vi "create io files.vi"(11 "path":path) -> (0 "interrupts.c":string, 2 "void init_ios(void)":string, 3 "defines":string)   [LabVIEW 2010]
uses:
  read_excel_values.llb/GetXL_CellValues_2D_String.vi
panel:
  out "error out":errorcluster
  # "Type: U8, I8, U16, I16, U32, I32, U64, I64, FLOAT"
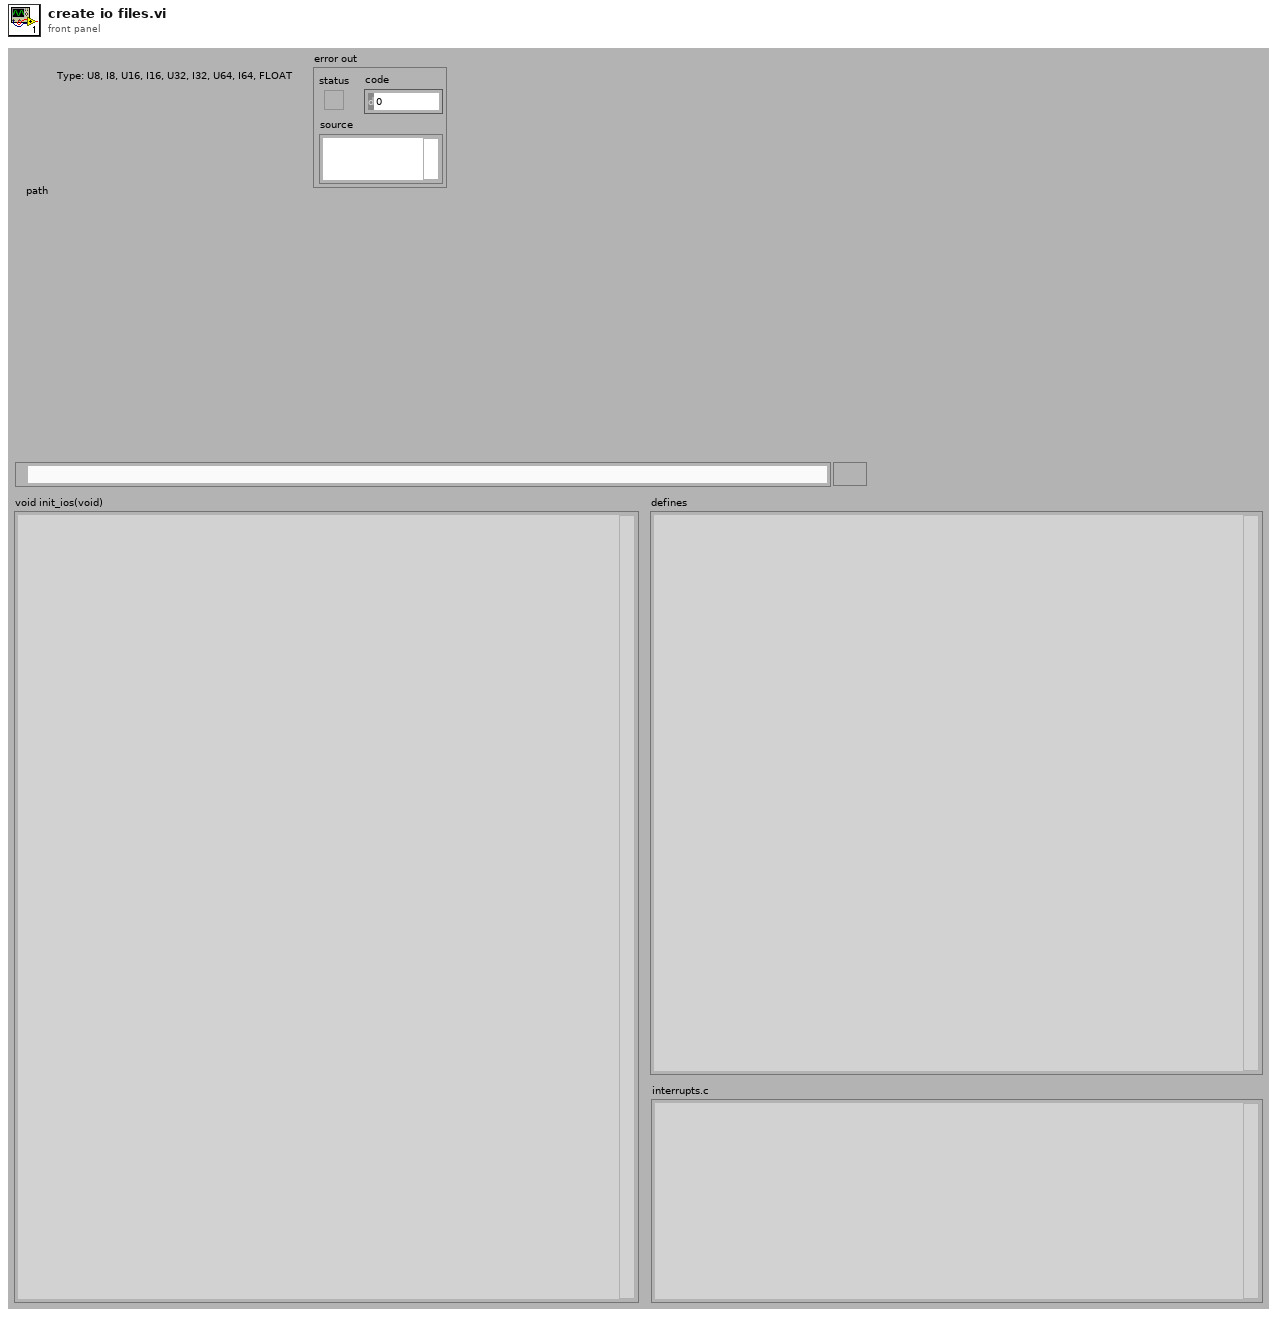
[diagram p1: front panel]
types:
  T1 = cluster{"Excel._Application":refnum<k7>, "Workbooks":refnum<k7>}
  T2 = cluster{"Excel._Application":refnum<k7>, "Workbooks":refnum<k7>, "Open":refnum<k7>}
  T3 = cluster{"Excel._Application":refnum<k7>, "Workbooks":refnum<k7>, "Open":refnum<k7>, "Worksheets":refnum<k7>, "Excel._Worksheet":refnum<k7>}
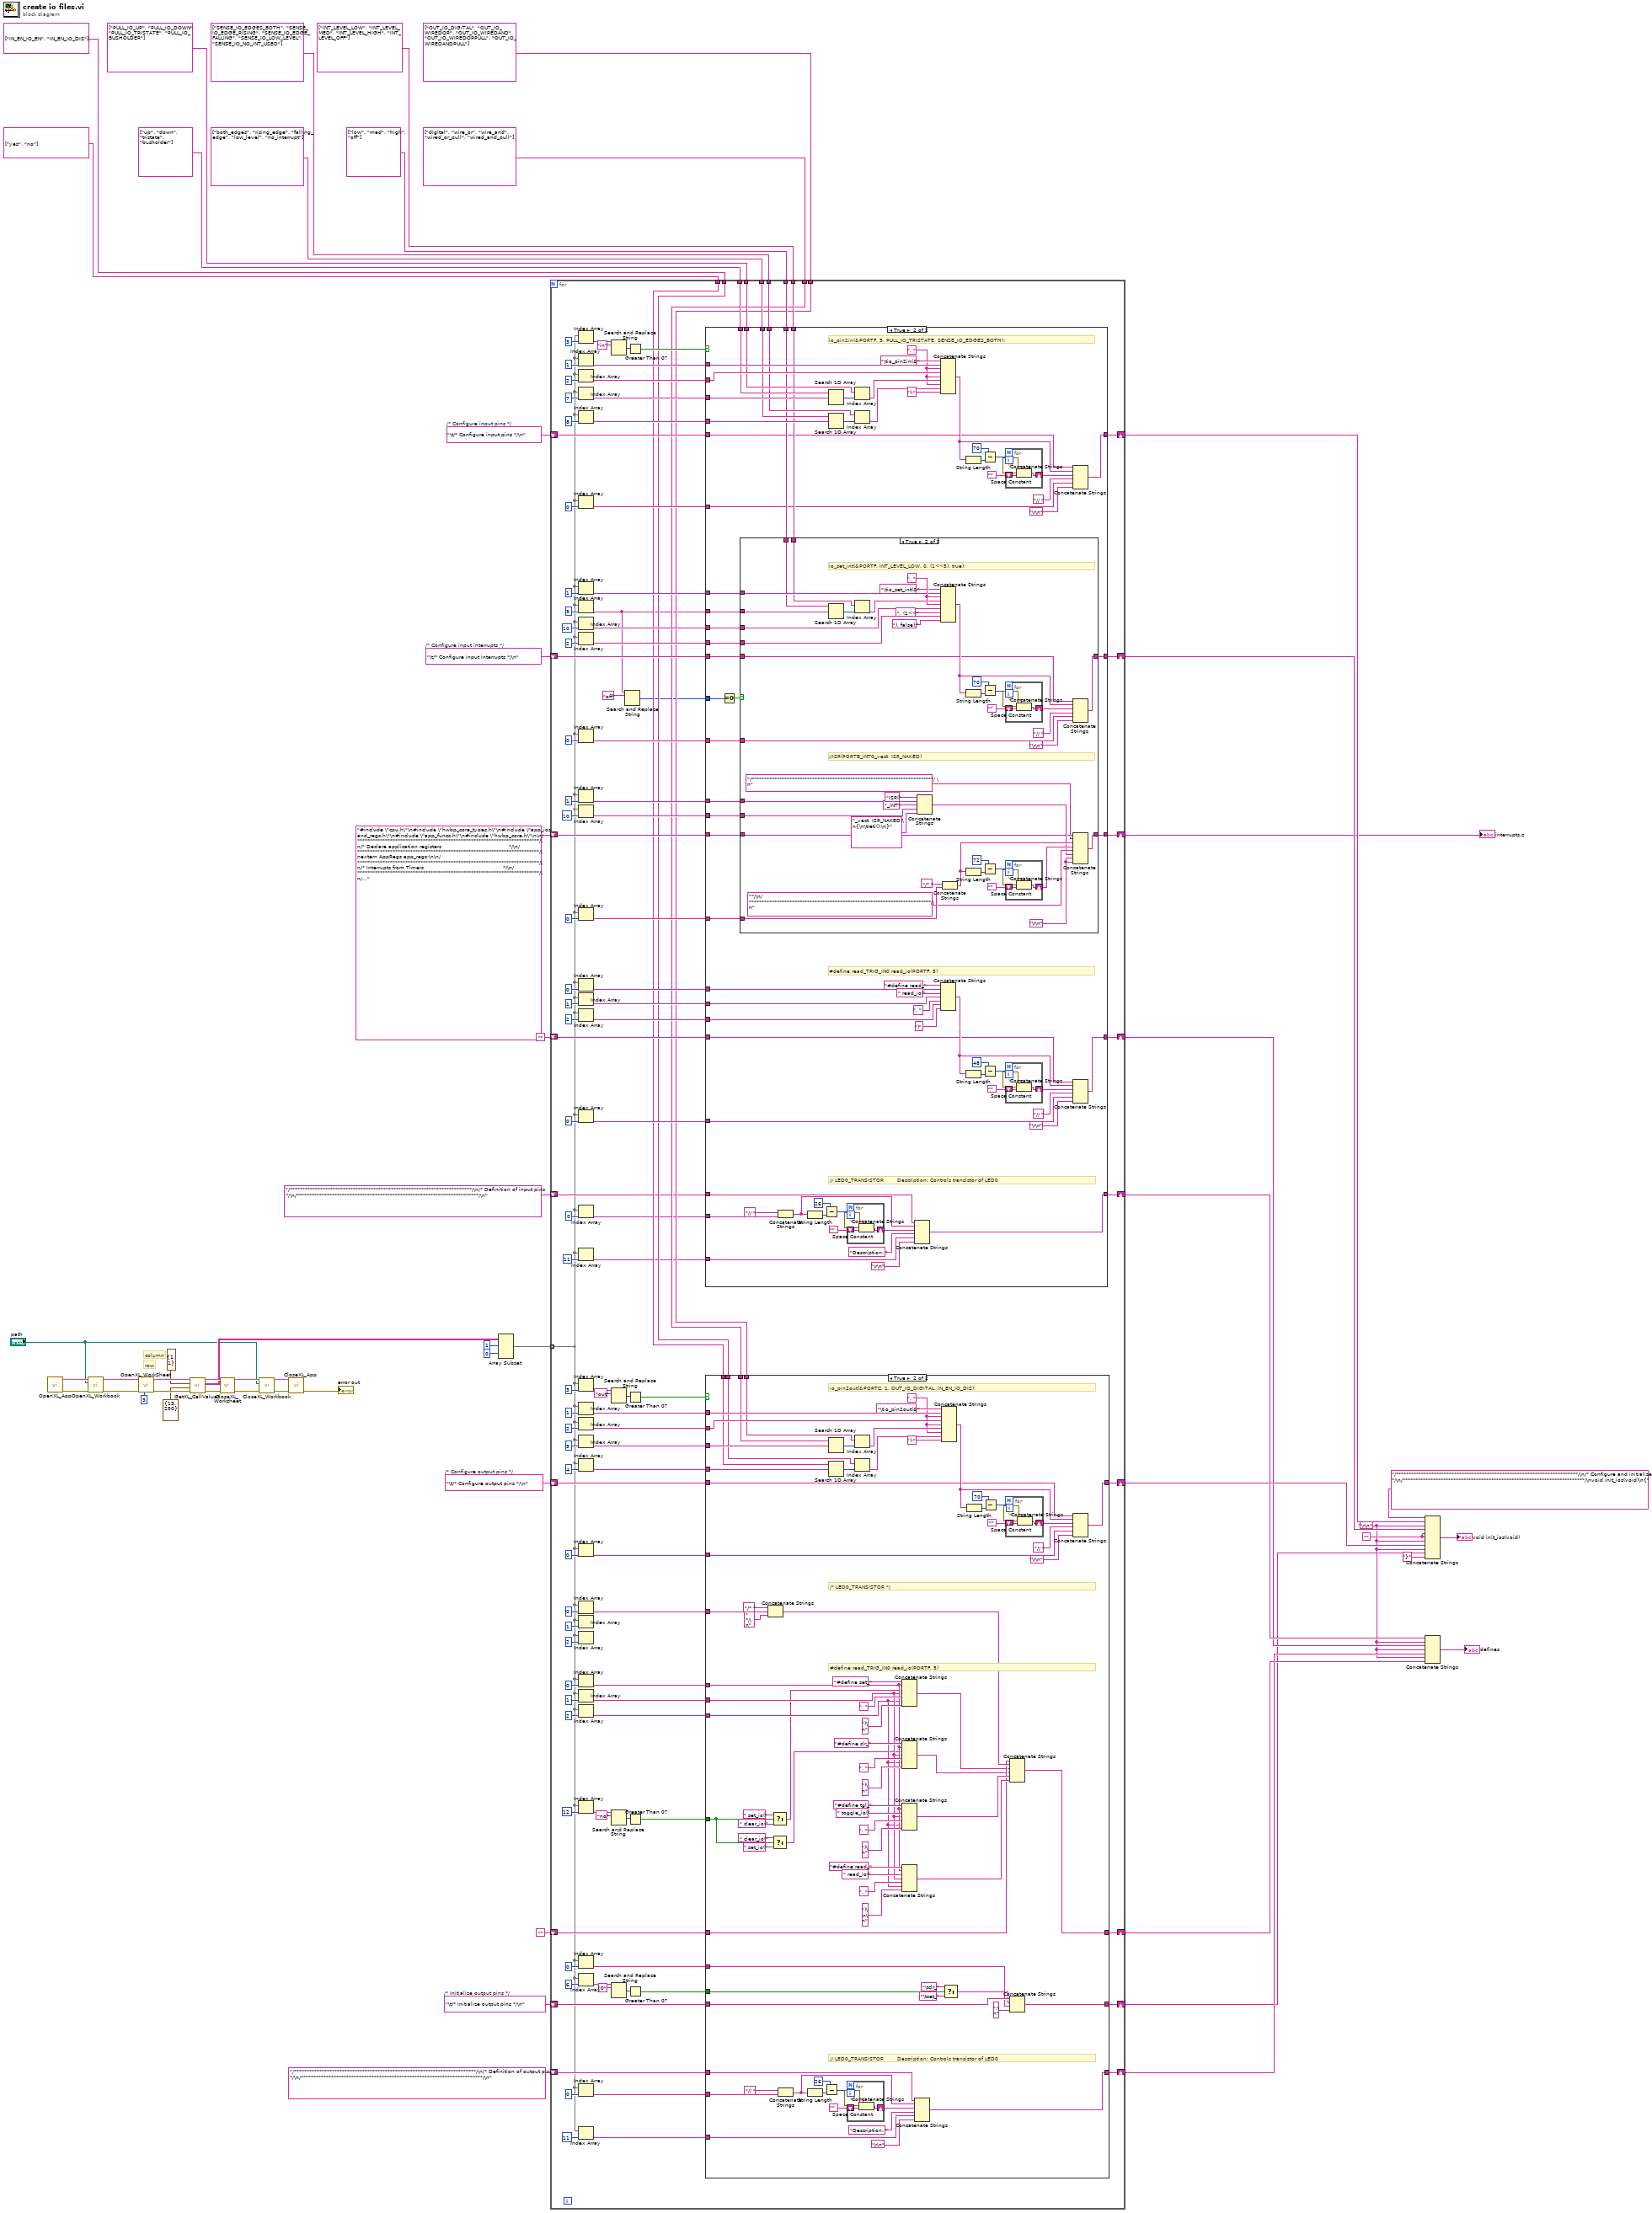
[diagram p0: block diagram]
diagram:
  w1 = ""
  w7 = "\t/* Configure input interrupts */\n"  # /* Configure input interrupts */
  w8 = "\t/* Configure output pins */\n"  # /* Configure output pins */
  w9 = "\t/* Configure input pins */\n"  # /* Configure input pins */
  w10 = "\t/* Initialize output pins */\n"  # /* Initialize output pins */
  w12 = "\r\n"
  # "row"
  # "column"
  n1 = call "OpenXL_App.vi"() -> ("error out"=w47:errorcluster, "Refnum Cluster"=w48:T1)  [unwired: 10 in]
  n2 = call "OpenXL_Workbook.vi"("error in"=w47, "path"="path", "Refnum Cluster In"=w48) -> ("error out"=w33:errorcluster, "Refnum Cluster Out"=w36:T2)  [unwired: 7 in]
  n3 = call "OpenXL_WorkSheet.vi"("Sheet"=3, "error in (no error)"=w33, "Refnum Cluster In"=w36) -> ("error out"=w54:errorcluster, "Refnum Cluster Out"=w55:T3)  [unwired: 7 in]
  n4 = call-poly "GetXL_CellValues.vi"("error in"=w54, "End"=cluster{"Column":i32, "Row":i32} {"Column"=13, "Row"=250}, "Start"=cluster{"Column":i32, "Row":i32} {"Column"=1, "Row"=1}, "Refnum Cluster In"=w55) -> ("error out"=w45:errorcluster, "data"=w40:string[][], "Refnum Cluster Out"=w46:T3)  [unwired: 5 in]
  n5 = call "CloseXL_Worksheet.vi"("error in (no error)"=w45, "Refnum Cluster In"=w46) -> ("error out"=w43:errorcluster, "Refnum Cluster Out"=w44:T2)  [unwired: 8 in]
  n6 = call "CloseXL_Workbook.vi"("error in (no error)"=w43, "path"="path", "Refnum Cluster In"=w44) -> ("error out"=w52:errorcluster, "Refnum Cluster Out"=w53:T1)  [unwired: 7 in]
  n7 = call "CloseXL_App.vi"("error in (no error)"=w52, "Refnum Cluster In"=w53) -> ("error out"=→"error out":errorcluster)  [unwired: 9 in]
  n8 = Array Subset(array=w40, index (row)=1 ("index"), index (col)=0 ("index")) -> (w37:string[][])  [unwired: 2 in]
  n9 = for {
    tunnel: w37 -> [w63] mode=indexing
    tunnel: string[] ["both_edges", "rising_edge", "falling_edge", "low_level", "no_interrupt"] -> [w155]
    tunnel: string[] ["up", "down", "tristate", "busholder"] -> [w159]
    shift-right: [w152] -> w23
    shift-left: w9 -> [w153]
    tunnel: string[] ["yes", "no"] -> [w95]
    tunnel: string[] ["IN_EN_IO_EN", "IN_EN_IO_DIS"] -> [w94]
    tunnel: string[] ["PULL_IO_UP", "PULL_IO_DOWN", "PULL_IO_TRISTATE", "PULL_IO_BUSHOLDER"] -> [w158]
    tunnel: string[] ["SENSE_IO_EDGES_BOTH", "SENSE_IO_EDGE_RISING", "SENSE_IO_EDGE_FALLING", "SENSE_IO_LOW_LEVEL", "SENSE_IO_NO_INT_USED"] -> [w154]
    tunnel: string[] ["low", "med", "high", "off"] -> [w142]
    tunnel: string[] ["INT_LEVEL_LOW", "INT_LEVEL_MED", "INT_LEVEL_HIGH", "INT_LEVEL_OFF"] -> [w141]
    tunnel: string[] ["digital", "wire_or", "wire_and", "wired_or_pull", "wired_and_pull"] -> [w92]
    tunnel: string[] ["OUT_IO_DIGITAL", "OUT_IO_WIREDOR", "OUT_IO_WIREDAND", "OUT_IO_WIREDORPULL", "OUT_IO_WIREDANDPULL"] -> [w93]
    shift-right: [w151] -> w24
    shift-left: w7 -> [w150]
    shift-right: [w129] -> w2
    shift-left: "#include \"cpu.h\"\n#include \"hwbp_core_types.h\"\n#include \"app_ios_and_regs.h\"\n#include \"app_funcs.h\"\n#include \"hwbp_core.h\"\n\n/************************************************************************/\n/* Declare application registers                                        */\n/************************************************************************/\nextern AppRegs app_regs;\n\n/************************************************************************/\n/* Interrupts from Timers                                               */\n/************************************************************************/\n// ISR(TCC0_OVF_vect, ISR_NAKED)\n// ISR(TCD0_OVF_vect, ISR_NAKED)\n// ISR(TCE0_OVF_vect, ISR_NAKED)\n// ISR(TCF0_OVF_vect, ISR_NAKED)\n// \n// ISR(TCC0_CCA_vect, ISR_NAKED)\n// ISR(TCD0_CCA_vect, ISR_NAKED)\n// ISR(TCE0_CCA_vect, ISR_NAKED)\n// ISR(TCF0_CCA_vect, ISR_NAKED)\n// \n// ISR(TCD1_OVF_vect, ISR_NAKED)\n// \n// ISR(TCD1_CCA_vect, ISR_NAKED)\n\n" -> [w130]
    shift-right: [w128] -> w14
    shift-left: "" -> [w127]
    shift-right: [w110] -> w19
    shift-left: w8 -> [w109]
    shift-right: [w89] -> w13
    shift-left: "/************************************************************************/\n/* Definition of output pins                                            */\n/************************************************************************/\n" -> [w88]
    shift-right: [w80] -> w11
    shift-left: "" -> [w87]
    shift-right: [w77] -> w15
    shift-left: "/************************************************************************/\n/* Definition of input pins                                             */\n/************************************************************************/\n" -> [w74]
    shift-right: [w72] -> w5
    shift-left: w10 -> [w71]
    n10 = Index Array(array=w63, index=3) -> (element=w168:string)
    n11 = Index Array(array=w63, index=1) -> (element=w164:string)
    n12 = Index Array(array=w63, index=2) -> (element=w162:string)
    n13 = Index Array(array=w63, index=7) -> (element=w160:string)
    n14 = Index Array(array=w63, index=8) -> (element=w156:string)
    n15 = Index Array(array=w63, index=0) -> (element=w135:string)
    n16 = Index Array(array=w63, index=1) -> (element=w144:string)
    n17 = Index Array(array=w63, index=9) -> (element=w58:string)
    n18 = Index Array(array=w63, index=10) -> (element=w149:string)
    n19 = Index Array(array=w63, index=2) -> (element=w146:string)
    n20 = Index Array(array=w63, index=0) -> (element=w134:string)
    n21 = Index Array(array=w63, index=1) -> (element=w139:string)
    n22 = Index Array(array=w63, index=10) -> (element=w137:string)
    n23 = Index Array(array=w63, index=0) -> (element=w131:string)
    n24 = Index Array(array=w63, index=0) -> (element=w122:string)
    n25 = Index Array(array=w63, index=1) -> (element=w124:string)
    n26 = Index Array(array=w63, index=2) -> (element=w119:string)
    n27 = Index Array(array=w63, index=0) -> (element=w126:string)
    n28 = Index Array(array=w63, index=3) -> (element=w98:string)
    n29 = Index Array(array=w63, index=1) -> (element=w102:string)
    n30 = Index Array(array=w63, index=2) -> (element=w104:string)
    n31 = Index Array(array=w63, index=5) -> (element=w106:string)
    n32 = Index Array(array=w63, index=4) -> (element=w108:string)
    n33 = Index Array(array=w63, index=0) -> (element=w112:string)
    n34 = Index Array(array=w63, index=0) -> (element=w116:string)
    n35 = Index Array(array=w63, index=1) -> ()  [unwired: 1 out]
    n36 = Index Array(array=w63, index=2) -> ()  [unwired: 1 out]
    n37 = Index Array(array=w63, index=0) -> (element=w84:string)
    n38 = Index Array(array=w63, index=1) -> (element=w86:string)
    n39 = Index Array(array=w63, index=2) -> (element=w81:string)
    n40 = Index Array(array=w63, index=12) -> (element=w60:string)
    n41 = Index Array(array=w63, index=0) -> (element=w65:string)
    n42 = Index Array(array=w63, index=6) -> (element=w68:string)
    n43 = Index Array(array=w63, index=0) -> (element=w90:string)
    n44 = Index Array(array=w63, index=11) -> (element=w113:string)
    n45 = Index Array(array=w63, index=0) -> (element=w76:string)
    n46 = Index Array(array=w63, index=11) -> (element=w75:string)
    n47 = Search and Replace String(input string=w168, search string="in") -> (number of replacements=w166:i32)  [unwired: 6 in, 3 out]
    n48 = Search and Replace String(input string=w98, search string="out") -> (number of replacements=w100:i32)  [unwired: 6 in, 3 out]
    n49 = Search and Replace String(input string=w60, search string="no") -> (number of replacements=w62:i32)  [unwired: 6 in, 3 out]
    n50 = Search and Replace String(input string=w68, search string="0") -> (number of replacements=w69:i32)  [unwired: 6 in, 3 out]
    n51 = Search and Replace String(input string=w58, search string="off") -> (number of replacements=w56:i32)  [unwired: 6 in, 3 out]
    n52 = Greater Than 0?(x=w166) -> (x > 0?=w165:bool)
    n53 = Greater Than 0?(x=w100) -> (x > 0?=w101:bool)
    n54 = Greater Than 0?(x=w62) -> (x > 0?=w59:bool)
    n55 = Greater Than 0?(x=w69) -> (x > 0?=w67:bool)
    n56 = case shown="True" w165 {
      tunnel: w164 -> [_ w338]
      tunnel: w162 -> [_ w337]
      tunnel: w160 -> [_ w335]
      tunnel: w159 -> [_ w334]
      tunnel: w158 -> [_ w333]
      tunnel: w156 -> [_ w329]
      tunnel: w155 -> [_ w328]
      tunnel: w154 -> [_ w327]
      tunnel: w153 -> [w266 w306]
      tunnel: [w266 w307] -> w152
      tunnel: w144 -> [_ w323]
      tunnel: w146 -> [_ w319]
      tunnel: w58 -> [_ w324]
      tunnel: w149 -> [_ w320]
      tunnel: w150 -> [w265 w303]
      tunnel: [w265 w304] -> w151
      tunnel: w142 -> [_ w322]
      tunnel: w141 -> [_ w321]
      tunnel: w139 -> [_ w318]
      tunnel: w137 -> [_ w317]
      tunnel: w135 -> [_ w309]
      tunnel: w134 -> [_ w305]
      tunnel: w130 -> [w264 w302]
      tunnel: [w264 w301] -> w129
      tunnel: w131 -> [_ w300]
      tunnel: w122 -> [_ w287]
      tunnel: w124 -> [_ w288]
      tunnel: w127 -> [w263 w289]
      tunnel: [w263 w290] -> w128
      tunnel: w126 -> [_ w297]
      tunnel: w119 -> [_ w284]
      tunnel: [w262 w272] -> w77
      tunnel: w76 -> [_ w271]
      tunnel: w75 -> [_ w270]
      tunnel: w74 -> [w262 w269]
      tunnel: w56 -> [_ w267]
      frame False {
      }
      frame True {
        w331 = ", " ("string")
        # "// LED0_TRANSISTOR        Description: Controls transistor of LED0"
        # "#define read_TRIG_IN0 read_io(PORTF, 5)"
        # "io_pin2in(&PORTF, 5, PULL_IO_TRISTATE, SENSE_IO_EDGES_BOTH);"
        n57 = Equal To 0?(x=w267) -> (x = 0?=w268:bool)
        n58 = case shown="True" w268 {
          tunnel: w324 -> [_ w382]
          tunnel: w323 -> [_ w380]
          tunnel: w322 -> [_ w378]
          tunnel: w321 -> [_ w377]
          tunnel: w320 -> [_ w375]
          tunnel: w319 -> [_ w373]
          tunnel: w318 -> [_ w368]
          tunnel: w317 -> [_ w367]
          tunnel: w305 -> [_ w365]
          tunnel: [w341 w357] -> w304
          tunnel: w303 -> [w341 w356]
          tunnel: w302 -> [w340 w343]
          tunnel: [w340 w355] -> w301
          tunnel: w300 -> [_ w348]
          frame False {
          }
          frame True {
            w344 = "\r\n"
            w383 = ", " ("string")
            # "//ISR(PORTB_INT0_vect, ISR_NAKED)"
            # "io_set_int(&PORTF, INT_LEVEL_LOW, 0, (1<<5), true);"
            n59 = Search 1D Array(1D array=w378, element=w382) -> (index of element=w381:i32)  [unwired: 1 in]
            n60 = Index Array(array=w377, index=w381) -> (element=w376:string)
            n61 = Concatenate Strings("ISR(" ("string"), w368, "_INT" ("string"), w367, "_vect, ISR_NAKED)\n{\n\treti();\n}" ("string")) -> (w345:string)
            n62 = Concatenate Strings("\tio_set_int(&" ("string"), w380, w383, w376, w383, w375, ", (1<<" ("string"), w373, "), false);" ("string")) -> (w358:string)
            n63 = Concatenate Strings("/* " ("string"), w348) -> (w347:string)
            n64 = String Length(string=w358) -> (length=w359:i32)
            n65 = String Length(string=w347) -> (length=w354:i32)
            n66 = Subtract(x=70, y=w359) -> (x-y=w361:i32)
            n67 = Subtract(x=72, y=w354) -> (x-y=w352:i32)
            n68 = for {
              N: w361 -> [_]
              shift-right: [w387] -> w363
              shift-left: "" -> [w389]
              n69 = call <vilib>:"Space Constant.vi"() -> ("String"=w388:string)
              n70 = Concatenate Strings(w388, w389) -> (w387:string)
            }
            n71 = for {
              N: w352 -> [_]
              shift-right: [w384] -> w350
              shift-left: "" -> [w386]
              n72 = call <vilib>:"Space Constant.vi"() -> ("String"=w385:string)
              n73 = Concatenate Strings(w385, w386) -> (w384:string)
            }
            n74 = Concatenate Strings(w356, w358, w363, "// " ("string"), w365, "\r\n") -> (w357:string)
            n75 = Concatenate Strings(w343, "/************************************************************************/ \n" ("string"), w347, w350, "*/\n/************************************************************************/\n" ("string"), w345, w344, w344) -> (w355:string)
          }
        }
        n76 = Concatenate Strings("// " ("string"), w271) -> (w281:string)
        n77 = String Length(string=w281) -> (length=w274:i32)
        n78 = Subtract(x=26, y=w274) -> (x-y=w276:i32)
        n79 = Search 1D Array(1D array=w334, element=w335) -> (index of element=w336:i32)  [unwired: 1 in]
        n80 = Search 1D Array(1D array=w328, element=w329) -> (index of element=w330:i32)  [unwired: 1 in]
        n81 = for {
          N: w276 -> [_]
          shift-right: [w390] -> w278
          shift-left: "" -> [w392]
          n82 = call <vilib>:"Space Constant.vi"() -> ("String"=w391:string)
          n83 = Concatenate Strings(w391, w392) -> (w390:string)
        }
        n84 = Index Array(array=w333, index=w336) -> (element=w332:string)
        n85 = Index Array(array=w327, index=w330) -> (element=w326:string)
        n86 = Concatenate Strings(w269, w281, w278, "Description: " ("string"), w270, "\r\n") -> (w272:string)
        n87 = Concatenate Strings("\tio_pin2in(&" ("string"), w338, w331, w337, w331, w332, w331, w326, ");" ("string")) -> (w311:string)
        n88 = Concatenate Strings("#define read_" ("string"), w287, " read_io(" ("string"), w288, ", " ("string"), w284, ")" ("string")) -> (w299:string)
        n89 = String Length(string=w311) -> (length=w316:i32)
        n90 = String Length(string=w299) -> (length=w291:i32)
        n91 = Subtract(x=70, y=w316) -> (x-y=w314:i32)
        n92 = Subtract(x=48, y=w291) -> (x-y=w293:i32)
        n93 = for {
          N: w314 -> [_]
          shift-right: [w396] -> w312
          shift-left: "" -> [w398]
          n94 = call <vilib>:"Space Constant.vi"() -> ("String"=w397:string)
          n95 = Concatenate Strings(w397, w398) -> (w396:string)
        }
        n96 = for {
          N: w293 -> [_]
          shift-right: [w393] -> w295
          shift-left: "" -> [w395]
          n97 = call <vilib>:"Space Constant.vi"() -> ("String"=w394:string)
          n98 = Concatenate Strings(w394, w395) -> (w393:string)
        }
        n99 = Concatenate Strings(w306, w311, w312, "// " ("string"), w309, "\r\n") -> (w307:string)
        n100 = Concatenate Strings(w289, w299, w295, "// " ("string"), w297, "\r\n") -> (w290:string)
      }
    }
    n101 = case shown="True" w101 {
      tunnel: w102 -> [_ w254]
      tunnel: w104 -> [_ w253]
      tunnel: w106 -> [_ w251]
      tunnel: w92 -> [_ w229]
      tunnel: w93 -> [_ w230]
      tunnel: w108 -> [_ w247]
      tunnel: w109 -> [w174 w234]
      tunnel: [w174 w235] -> w110
      tunnel: w112 -> [_ w237]
      tunnel: w116 -> [_ w233]
      tunnel: w113 -> [_ w216]
      tunnel: w95 -> [_ w227]
      tunnel: w94 -> [_ w228]
      tunnel: w90 -> [_ w225]
      tunnel: w88 -> [w173 w215]
      tunnel: [w173 w214] -> w89
      tunnel: w84 -> [_ w199]
      tunnel: w86 -> [_ w198]
      tunnel: w87 -> [w172 w192]
      tunnel: w81 -> [_ w197]
      tunnel: [w172 w193] -> w80
      tunnel: w71 -> [w171 w185]
      tunnel: [w171 w188] -> w72
      tunnel: w67 -> [_ w191]
      tunnel: w65 -> [_ w184]
      tunnel: w59 -> [_ w177]
      frame False {
      }
      frame True {
        w249 = ", " ("string")
        # "// LED0_TRANSISTOR        Description: Controls transistor of LED0"
        # "#define read_TRIG_IN0 read_io(PORTF, 5)"
        # "/* LED0_TRANSISTOR */"
        # "io_pin2out(&PORTC, 1, OUT_IO_DIGITAL, IN_EN_IO_DIS);"
        n102 = Concatenate Strings("/* " ("string"), w233, " */\n" ("string")) -> (w196:string)
        n103 = Select(t=" set_io(", s=w177, f=" clear_io(") -> (s? t:f=w176:string)
        n104 = Select(t=" clear_io(", s=w177, f=" set_io(") -> (s? t:f=w175:string)
        n105 = Concatenate Strings("// " ("string"), w225) -> (w217:string)
        n106 = String Length(string=w217) -> (length=w224:i32)
        n107 = Subtract(x=26, y=w224) -> (x-y=w222:i32)
        n108 = Search 1D Array(1D array=w229, element=w251) -> (index of element=w252:i32)  [unwired: 1 in]
        n109 = Search 1D Array(1D array=w227, element=w247) -> (index of element=w248:i32)  [unwired: 1 in]
        n110 = for {
          N: w222 -> [_]
          shift-right: [w256] -> w220
          shift-left: "" -> [w258]
          n111 = call <vilib>:"Space Constant.vi"() -> ("String"=w257:string)
          n112 = Concatenate Strings(w257, w258) -> (w256:string)
        }
        n113 = Index Array(array=w230, index=w252) -> (element=w250:string)
        n114 = Index Array(array=w228, index=w248) -> (element=w246:string)
        n115 = Concatenate Strings("#define set_" ("string"), w199, w176, w198, ", " ("string"), w197, ")\n" ("string")) -> (w189:string)
        n116 = Concatenate Strings("#define clr_" ("string"), w199, w175, w198, ", " ("string"), w197, ")\n" ("string")) -> (w190:string)
        n117 = Concatenate Strings("#define tgl_" ("string"), w199, " toggle_io(" ("string"), w198, ", " ("string"), w197, ")\n" ("string")) -> (w195:string)
        n118 = Concatenate Strings("#define read_" ("string"), w199, " read_io(" ("string"), w198, ", " ("string"), w197, ")\n\n" ("string")) -> (w194:string)
        n119 = Concatenate Strings(w215, w217, w220, "Description: " ("string"), w216, "\r\n") -> (w214:string)
        n120 = Concatenate Strings("\tio_pin2out(&" ("string"), w254, w249, w253, w249, w250, w249, w246, ");" ("string")) -> (w239:string)
        n121 = Select(t="\tclr_", s=w191, f="\tset_") -> (s? t:f=w183:string)
        n122 = String Length(string=w239) -> (length=w244:i32)
        n123 = Subtract(x=70, y=w244) -> (x-y=w242:i32)
        n124 = for {
          N: w242 -> [_]
          shift-right: [w259] -> w240
          shift-left: "" -> [w261]
          n125 = call <vilib>:"Space Constant.vi"() -> ("String"=w260:string)
          n126 = Concatenate Strings(w260, w261) -> (w259:string)
        }
        n127 = Concatenate Strings(w192, w196, w189, w190, w195, w194) -> (w193:string)
        n128 = Concatenate Strings(w185, w183, w184, ";\n" ("string")) -> (w188:string)
        n129 = Concatenate Strings(w234, w239, w240, "// " ("string"), w237, "\r\n") -> (w235:string)
      }
    }
  }
  "interrupts.c" <- w2
  n130 = Concatenate Strings("/************************************************************************/\n/* Configure and initialize IOs                                         */\n/************************************************************************/\nvoid init_ios(void)\n{", w23, w12, w24, w1, w1, w12, w19, w12, w5, "}") -> (→"void init_ios(void)":string)
  n131 = Concatenate Strings(w15, w12, w14, w12, w13, w12, w11) -> (→"defines":string)
